vi "Sched and Tubes.vi"(1 "Schedule":T1, 2 "Tube Type":T4, 8 "Error In":errorcluster, 10 "Preselected sched name":string, 11 "Preselected sched":string) -> (0 "Error Out":errorcluster)   [LabVIEW 2023]
uses:
  Schedule.ctl
  Tubes.ctl
  Schedule Name.ctl
  Params.ctl
  QSM - Editor/Controls/State Machine Message.ctl
  QSM - Editor/Controls/Message Queue Element Position.ctl
  QSM - Editor/QSM - Editor.lvlib
panel:
  out "SchedNames":string[](array[string])
  out "SchedNames[]":string[](array[string])
  in  "Tab Control":enum32{"Schedule", "Tubes"}(tab)
  in  "LOAD STEP VAL":bool
  in  "Schedule Name":string
  in  "Sched#":u16(ring) items=["", "Sched1", "Sched2", "Sched3", "Sched4", "Sched5", "Sched6", "Sched7", "Sched8", "Sched9", "Sched10", "Sched11", "Sched12", "Sched13", "Sched14", "Sched15", "Sched16", "Sched17", "Sched18", "Sched19", "Sched20", "Sched21", "Sched22", "Sched23", "Sched24", "Sched25", "Sched26", "Sched27", "Sched28", "Sched29", "Sched30", "Sched31", "Sched32", "Sched33", "Sched34", "Sched35", "Sched36", "Sched37", "Sched38", "Sched39", "Sched40", "Sched41", "Sched42", "Sched43", "Sched44", "Sched45", "Sched46", "Sched47", "Sched48", "Sched49", "Sched50", "Sched51", "Sched52", "Sched53", "Sched54", "Sched55", "Sched56", "Sched57", "Sched58", "Sched59", "Sched60", "Sched61", "Sched62", "Sched63", "Sched64", "Sched65", "Sched66", "Sched67", "Sched68", "Sched69", "Sched70", "Sched71", "Sched72", "Sched73", "Sched74", "Sched75", "Sched76", "Sched77", "Sched78", "Sched79", "Sched80"]
  in  "Load":bool
  out "Schedule Filename":T2
  in  "Save As\nSched":bool
  in  "Zero Sched":bool
  in  "Insert Step":bool
  in  "Delete Step":bool
  in  "Copy Step":bool
  in  "Paste Step":bool
  in  "stop":bool
  in  "stop 2":bool
  in  "Tube Save":bool
  in  "Sched 61-80":T3
  in  "Sched 31-60":T3
  in  "Sched 1-30":T3
  in  "Tube Values":T5
  out "Copied Row":string[](array[string])
  # "--SCHEDULE & TUBE EDITOR--"
  # "** Select tabs at the top to switch between tube & schedule editors"
  # "** If changes are made, please make sure to select the correct schedule and press the 'SAVE AS SCHED' button.\nClosing this screen without saving changes, will result in changes being lost."
  # "** Select tabs at the top to switch between tube & schedule editors"
  # "** To select a tube for editing, double click the desired tube inside the 'Tube Type' Table.\nTo save changed values, the 'SAVE' button must be selected on this screen next to the 'Tube Values' display.\nFailure to save before closing will result in loss of changes."
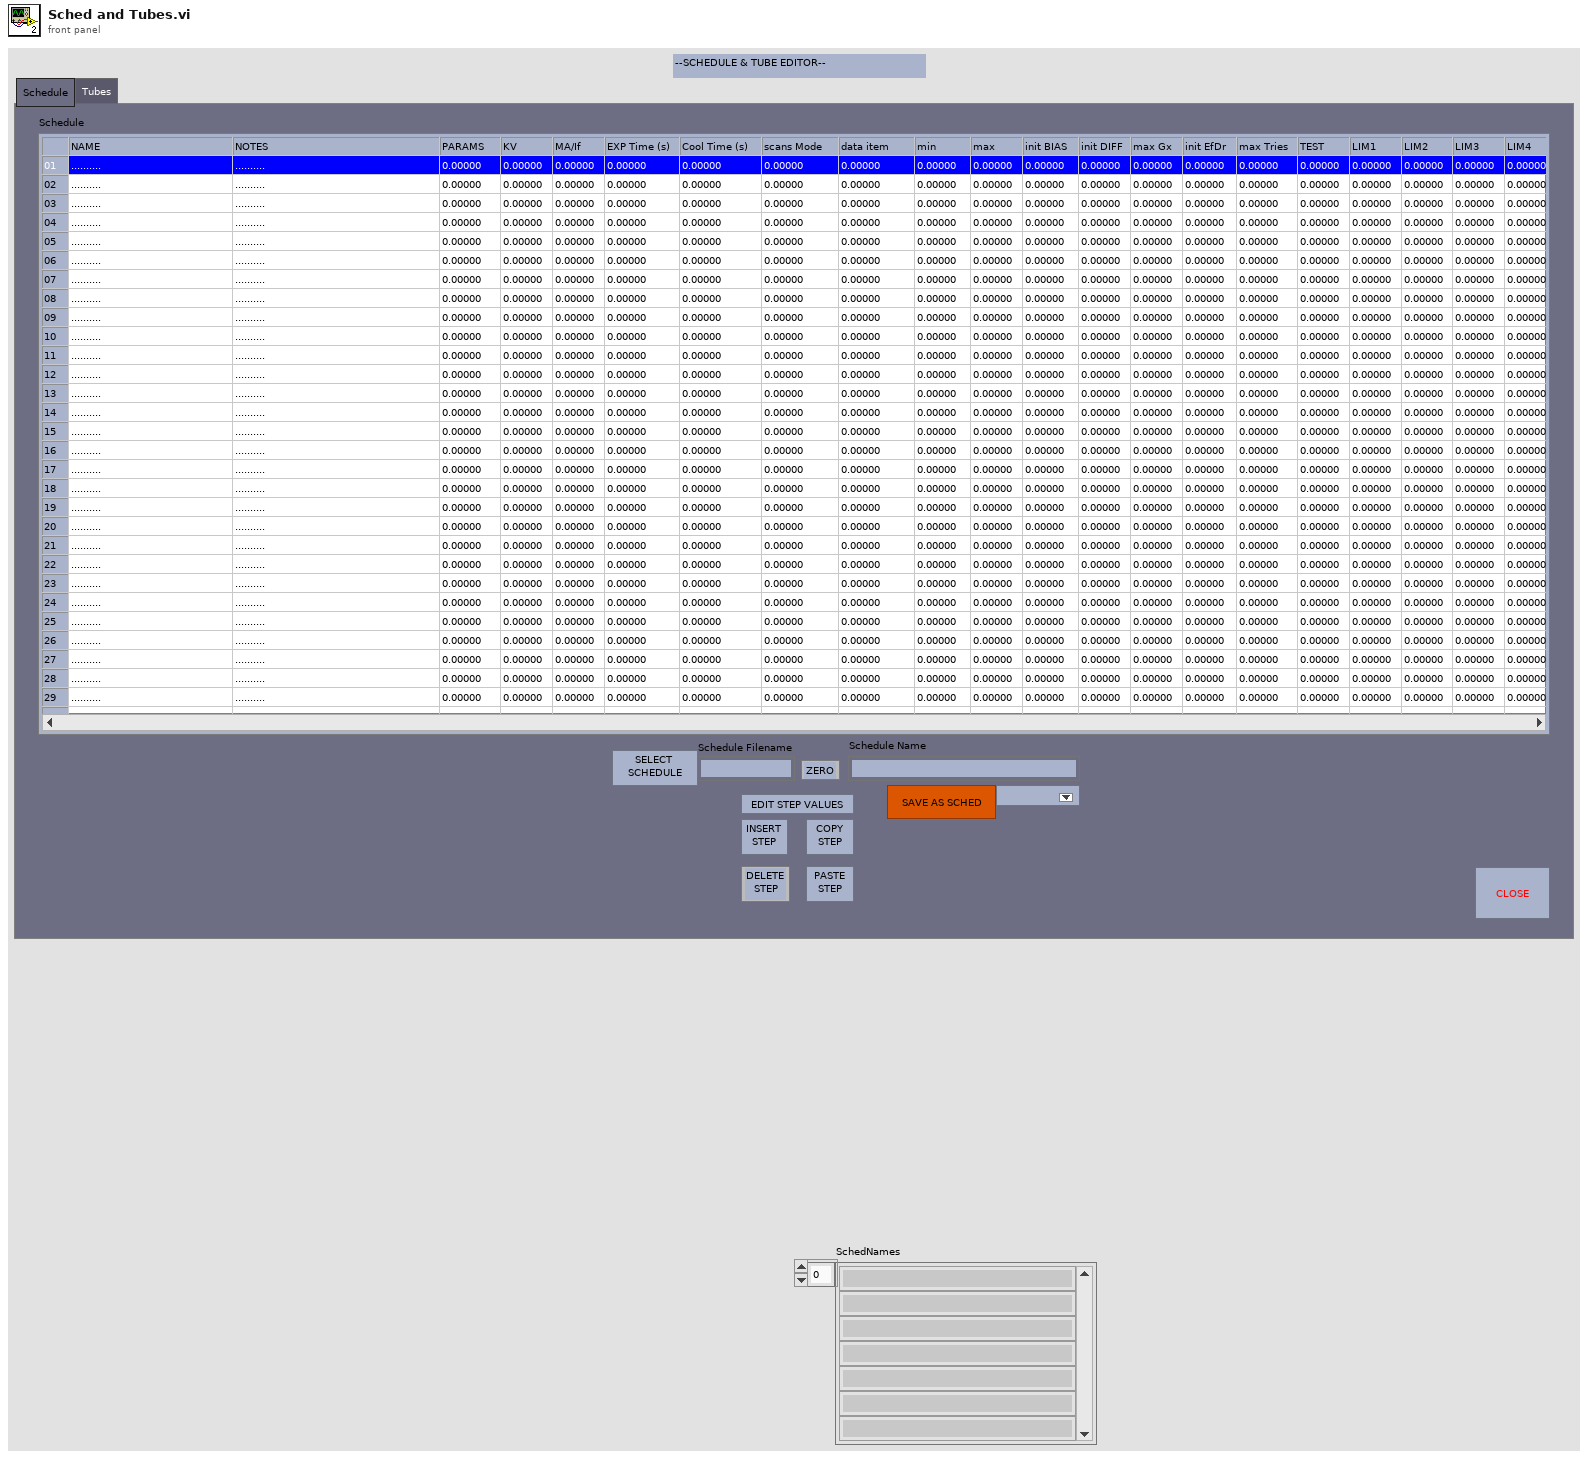
[diagram p1: front panel]
types:
  T1 = typedef "Schedule.ctl" = i32
  T2 = typedef "Schedule Name.ctl" = string
  T3 = typedef "Params.ctl" = cluster{"Boolean":bool, "Boolean 2":bool, "Boolean 3":bool, "Boolean 4":bool, "Boolean 5":bool, "Boolean 6":bool, "Boolean 7":bool, "Boolean 8":bool, "Boolean 9":bool, "Boolean 10":bool, "Boolean 11":bool, "Boolean 12":bool, "Boolean 13":bool, "Boolean 14":bool, "Boolean 15":bool, "Boolean 16":bool, "Boolean 17":bool, "Boolean 18":bool, "Boolean 19":bool, "Boolean 20":bool, "Boolean 21":bool, "Boolean 22":bool, "Boolean 23":bool, "Boolean 24":bool, "Boolean 25":bool, "Boolean 26":bool, "Boolean 27":bool, "Boolean 28":bool, "Boolean 29":bool, "Boolean 30":bool, "Boolean 31":bool, "Boolean 32":bool}
  T4 = typedef "Tubes.ctl" = i32
  T5 = cluster{"Tube Name":string, "T0":dbl, "RTC":dbl, "HS":dbl, "T100":dbl, "AP%":dbl}
  T6 = typedef "QSM - Editor.lvlib/State Machine Message.ctl" = enum16{"Initialize", "Handle Error", "Load", "Zero", "Insert", "Delete", "Copy", "Paste", "Save Sched", "Load Step Vals", "Tubes Tab", "Tube Select", "Tube Save", "Exit"}
  T7 = typedef "QSM - Editor.lvlib/Message Queue Element Position.ctl" = enum16{"Front", "Back"}
  T8 = cluster{"Boolean array[0]":bool, "Boolean array[1]":bool, "Boolean array[2]":bool, "Boolean array[3]":bool, "Boolean array[4]":bool, "Boolean array[5]":bool, "Boolean array[6]":bool, "Boolean array[7]":bool, "Boolean array[8]":bool, "Boolean array[9]":bool, "Boolean array[10]":bool, "Boolean array[11]":bool, "Boolean array[12]":bool, "Boolean array[13]":bool, "Boolean array[14]":bool, "Boolean array[15]":bool, "Boolean array[16]":bool, "Boolean array[17]":bool, "Boolean array[18]":bool, "Boolean array[19]":bool, "Boolean array[20]":bool, "Boolean array[21]":bool, "Boolean array[22]":bool, "Boolean array[23]":bool, "Boolean array[24]":bool, "Boolean array[25]":bool, "Boolean array[26]":bool, "Boolean array[27]":bool, "Boolean array[28]":bool, "Boolean array[29]":bool, "Boolean array[30]":bool, "Boolean array[31]":bool}
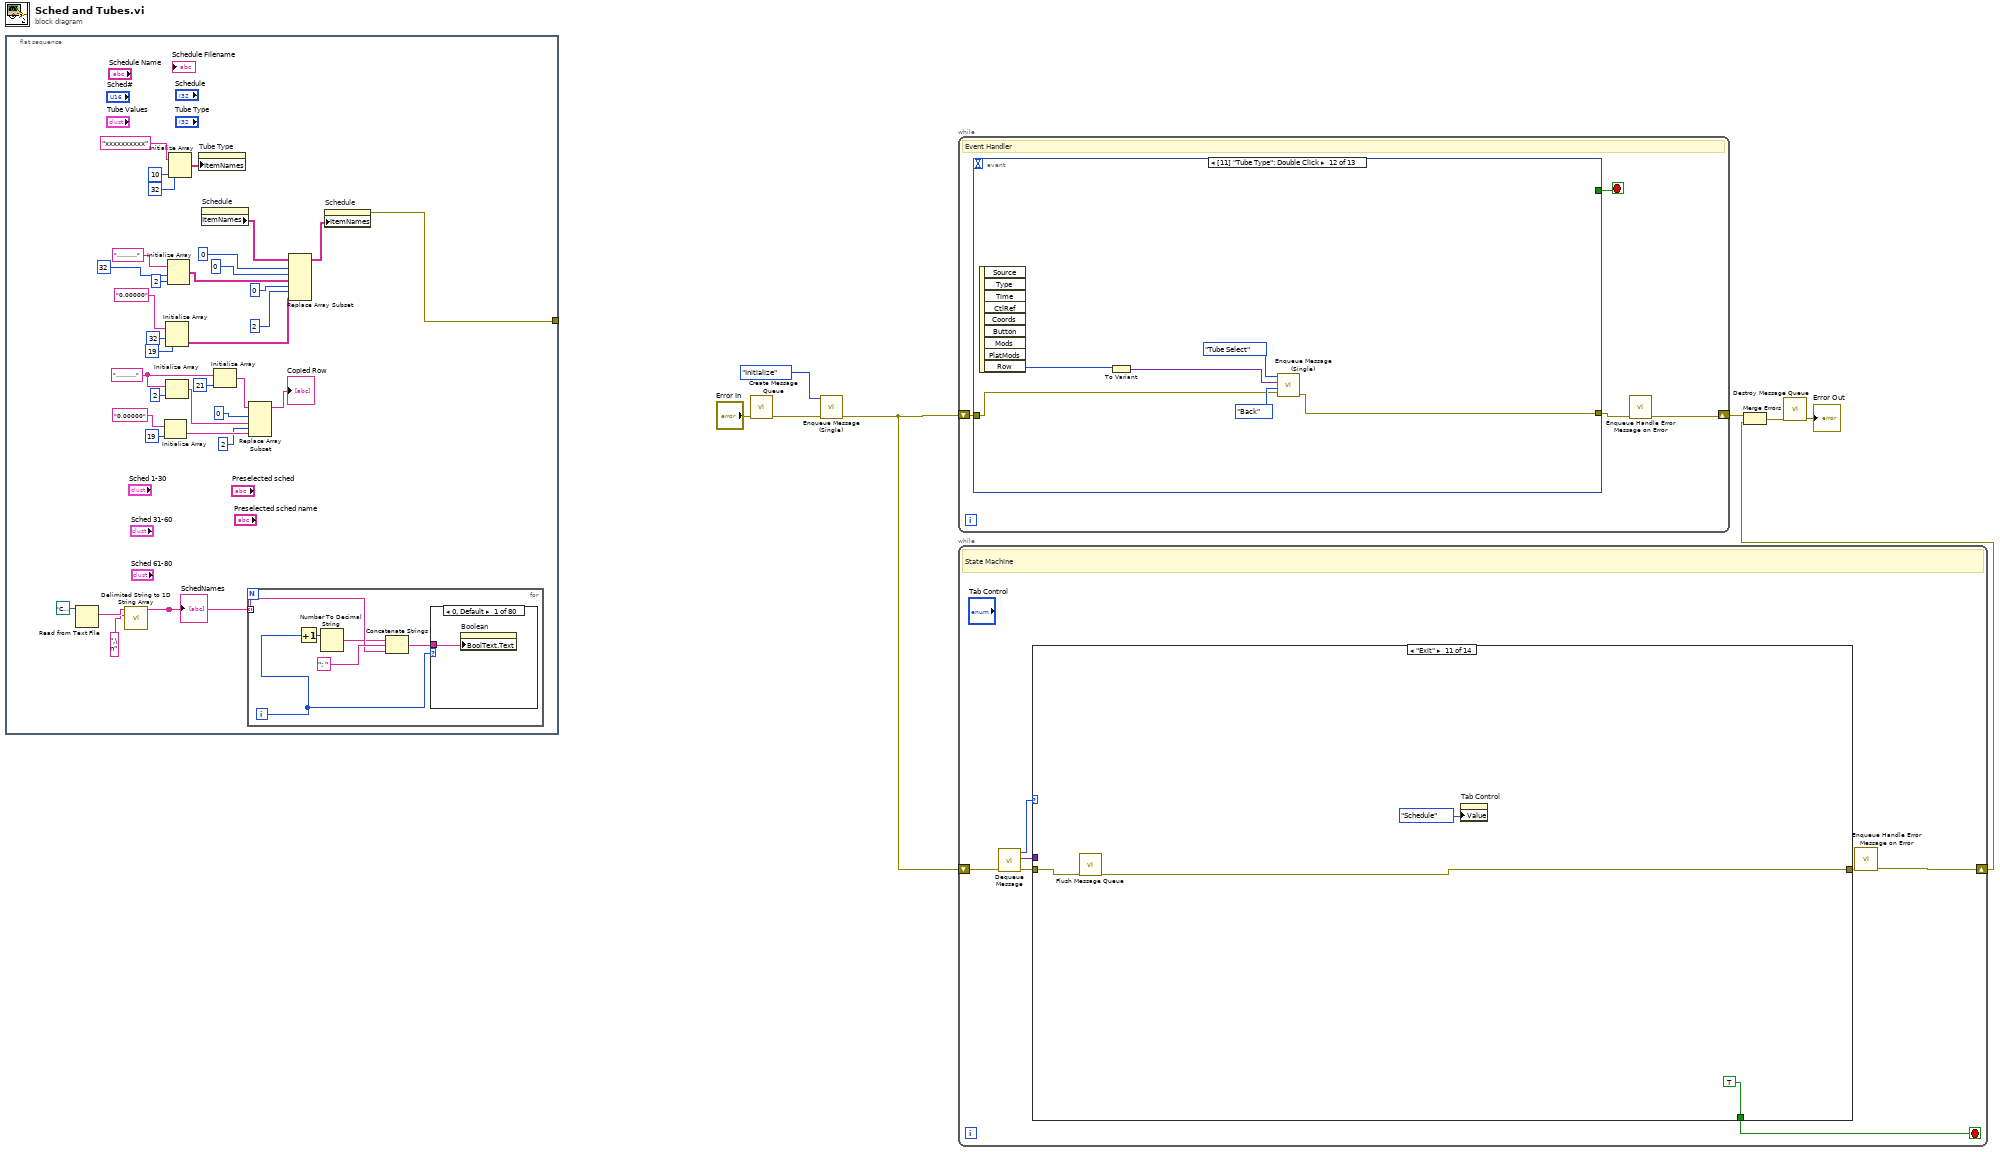
[diagram p0: block diagram]
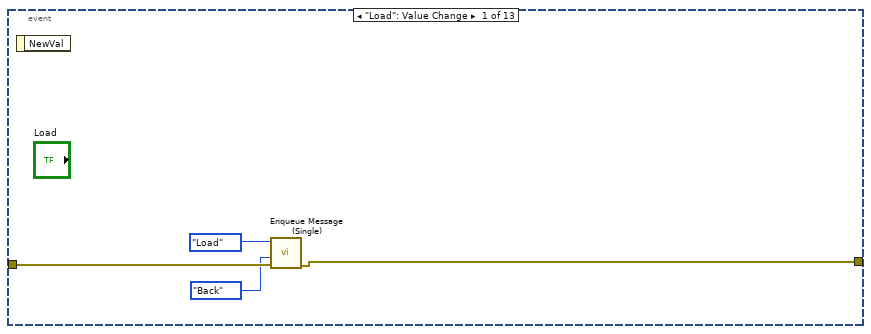
[diagram p2: hidden frame]
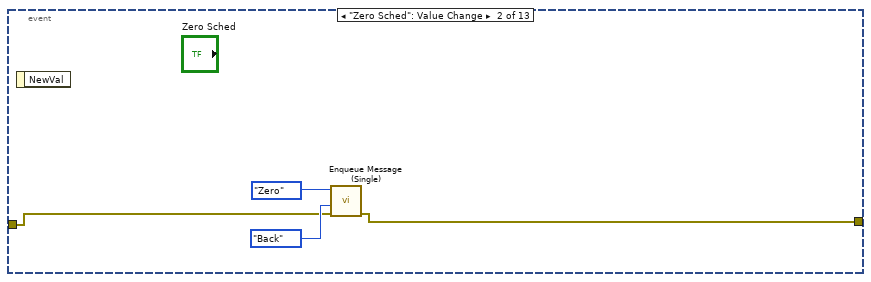
[diagram p3: hidden frame]
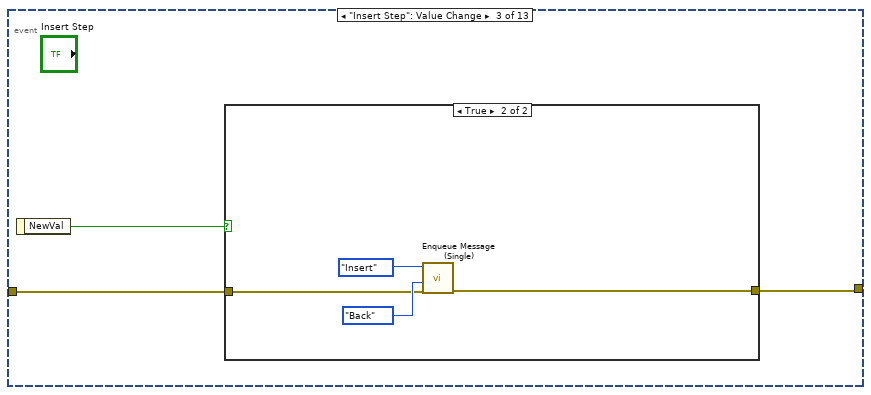
[diagram p4: hidden frame]
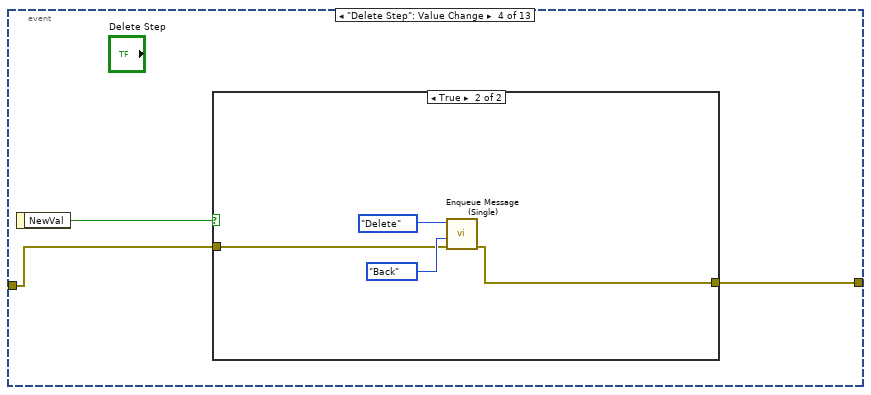
[diagram p6: hidden frame]
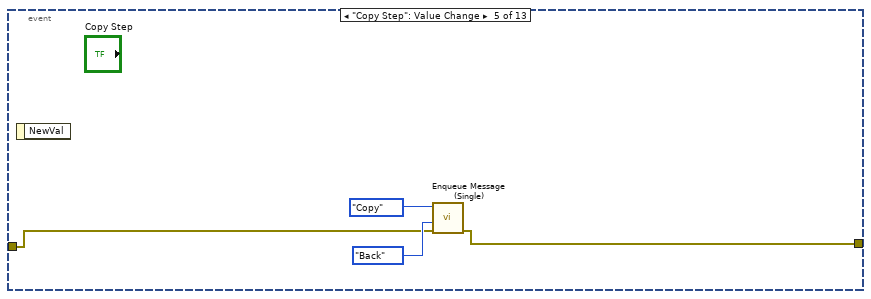
[diagram p8: hidden frame]
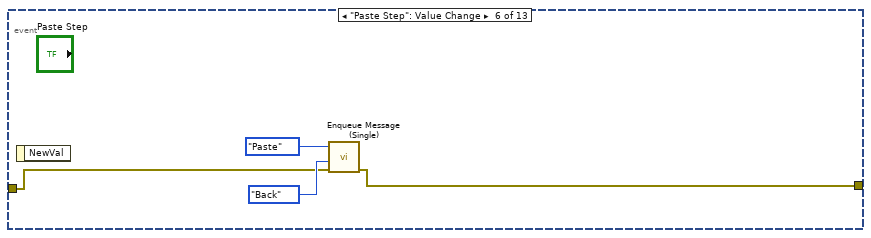
[diagram p9: hidden frame]
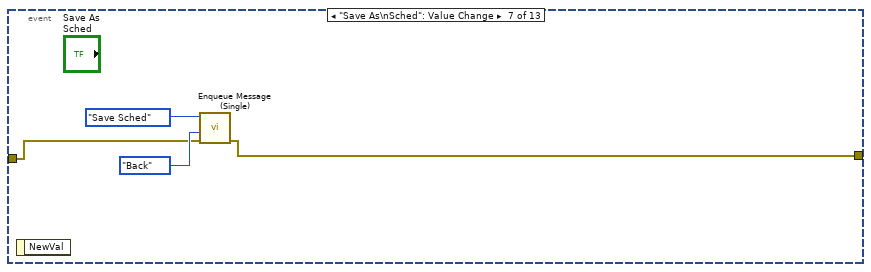
[diagram p10: hidden frame]
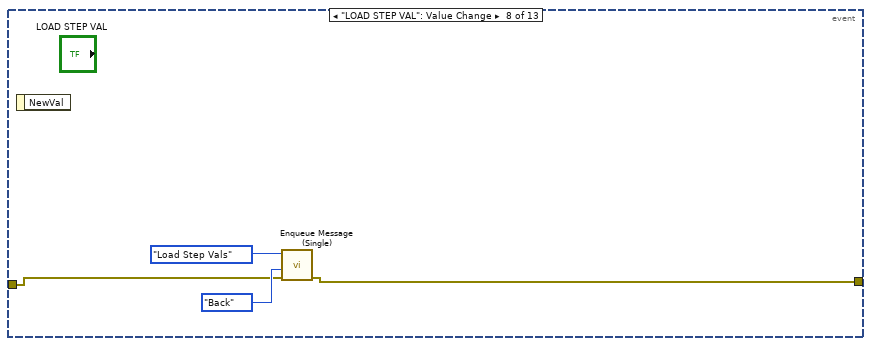
[diagram p11: hidden frame]
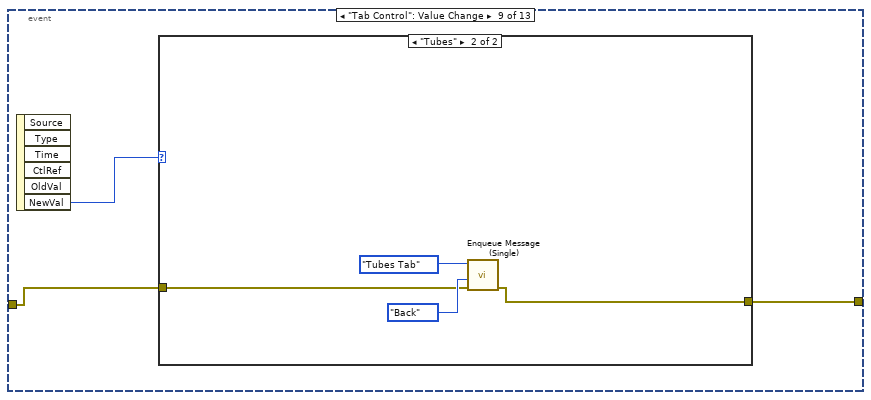
[diagram p12: hidden frame]
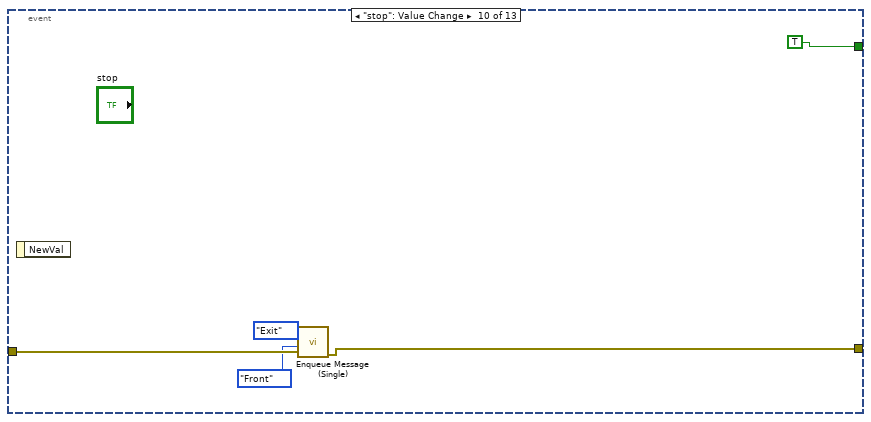
[diagram p14: hidden frame]
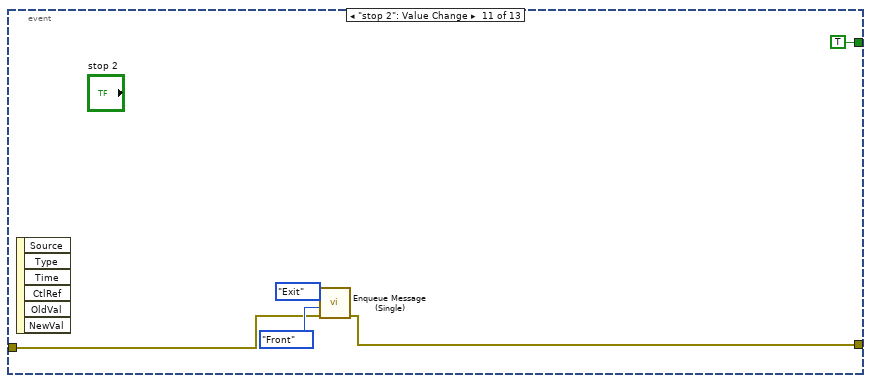
[diagram p15: hidden frame]
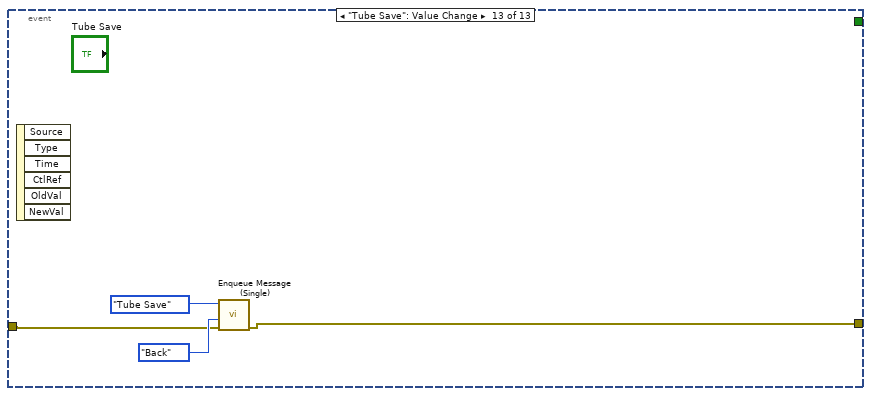
[diagram p16: hidden frame]
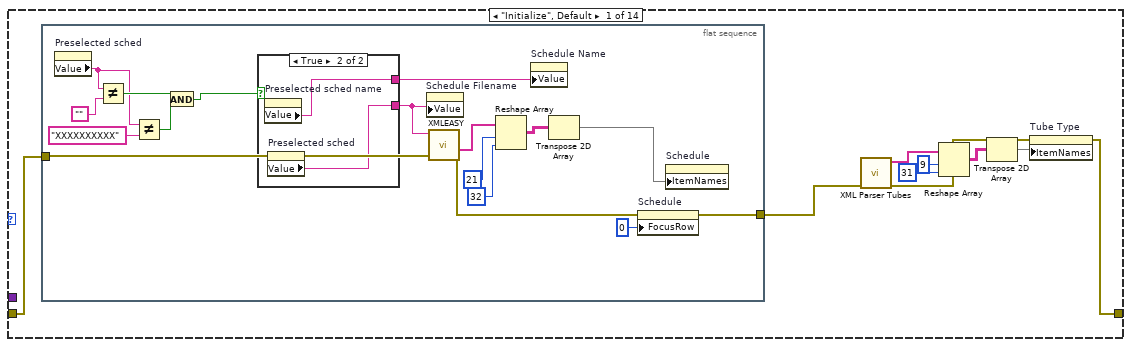
[diagram p17: hidden frame]
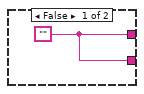
[diagram p18: hidden frame]
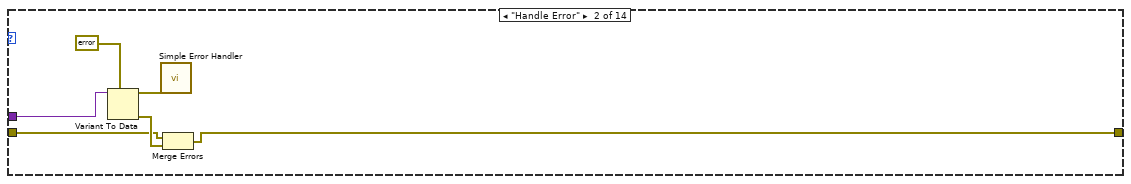
[diagram p19: hidden frame]
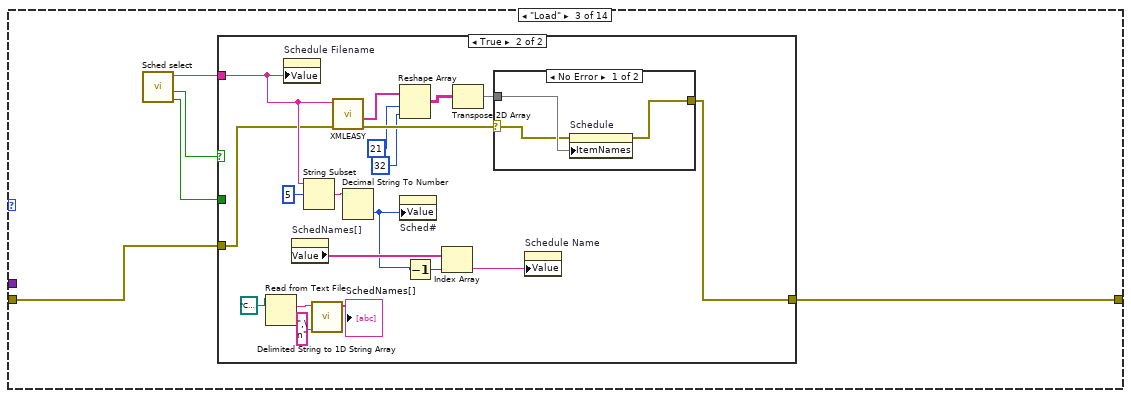
[diagram p20: hidden frame]
diagram:
  n1 = flat-sequence {
    tunnel: [w13] -> _
    frame #0 {
      w19 = ".........."
      n2 = Read from Text File(file (use dialog)=path "C:/Users/Public/Documents/Grid2093/SCHEDS/SchedNames.txt") -> (text=w11:string)  [unwired: 3 in, 3 out]
      n3 = call <vilib>:"Delimited String to 1D String Array.vi"("delimiter"=",\n", "delimited string"=w11) -> ("string array"=w12:string[])  [unwired: 9 in]
      "SchedNames" <- w12
      n4 = Initialize Array("0.00000", 19 ("dimension size")) -> (w23:string[])
      n5 = Initialize Array("0.00000", 32 ("dimension size"), 19 ("dimension size")) -> (w38:string[][])
      n6 = Initialize Array(w19, 2 ("dimension size")) -> (w22:string[])
      n7 = Initialize Array("..........", 32 ("dimension size"), 2 ("dimension size")) -> (w37:string[][])
      n8 = Initialize Array("xxxxxxxxxx", 32 ("dimension size"), 10 ("dimension size")) -> (w39:string[][])
      n9 = property on="Tube Type" class="MCListbox (strict)"("ItemNames"=w39) -> ()  [unwired: 2 in, 2 out]
      n10 = property on="Schedule" class="MCListbox (strict)"() -> ("ItemNames"=w25:string[][])  [unwired: 2 in, 2 out]
      n11 = Initialize Array(w19, 21 ("dimension size")) -> (w24:string[])
      n12 = for {
        tunnel: w12 -> [w47] mode=indexing
        i -> [w44]
        n13 = Increment(x=w44) -> (x+1=w45:i32)
        n14 = Number To Decimal String(number=w45) -> (decimal integer string=w46:string)  [unwired: 1 in]
        n15 = Concatenate Strings(w46, ": " ("string"), w47) -> (w43:string)
        n16 = case shown="0, Default" w44 {
          tunnel: w43 -> [w49 w50 w51 w52 w53 w54 w55 w56 w57 w58 w59 w60 w61 w62 w63 w64 w65 w66 w67 w68 w69 w70 w71 w72 w73 w74 w75 w76 w77 w78 w79 w80 w81 w82 w83 w84 w85 w86 w87 w88 w89 w90 w91 w92 w93 w94 w95 w96 w97 w98 w99 w100 w101 w102 w103 w104 w105 w106 w107 w108 w109 w110 w111 w112 w113 w114 w115 w116 w117 w118 w119 w120 w121 w122 w123 w124 w125 w126 w127 w128]
          frame 0, Default {
            n17 = property on="Boolean" class="Bool (strict)"("BoolText.Text"=w49) -> ()  [unwired: 2 in, 2 out]
          }
          frame 1 {
            n18 = property on="Boolean 2" class="Bool (strict)"("BoolText.Text"=w50) -> ()  [unwired: 2 in, 2 out]
          }
          frame 2 {
            n19 = property on="Boolean 3" class="Bool (strict)"("BoolText.Text"=w51) -> ()  [unwired: 2 in, 2 out]
          }
          frame 3 {
            n20 = property on="Boolean 4" class="Bool (strict)"("BoolText.Text"=w52) -> ()  [unwired: 2 in, 2 out]
          }
          frame 4 {
            n21 = property on="Boolean 5" class="Bool (strict)"("BoolText.Text"=w53) -> ()  [unwired: 2 in, 2 out]
          }
          frame 5 {
            n22 = property on="Boolean 6" class="Bool (strict)"("BoolText.Text"=w54) -> ()  [unwired: 2 in, 2 out]
          }
          frame 6 {
            n23 = property on="Boolean 7" class="Bool (strict)"("BoolText.Text"=w55) -> ()  [unwired: 2 in, 2 out]
          }
          frame 7 {
            n24 = property on="Boolean 8" class="Bool (strict)"("BoolText.Text"=w56) -> ()  [unwired: 2 in, 2 out]
          }
          frame 8 {
            n25 = property on="Boolean 9" class="Bool (strict)"("BoolText.Text"=w57) -> ()  [unwired: 2 in, 2 out]
          }
          frame 9 {
            n26 = property on="Boolean 10" class="Bool (strict)"("BoolText.Text"=w58) -> ()  [unwired: 2 in, 2 out]
          }
          frame 10 {
            n27 = property on="Boolean 11" class="Bool (strict)"("BoolText.Text"=w59) -> ()  [unwired: 2 in, 2 out]
          }
          frame 11 {
            n28 = property on="Boolean 12" class="Bool (strict)"("BoolText.Text"=w60) -> ()  [unwired: 2 in, 2 out]
          }
          frame 12 {
            n29 = property on="Boolean 13" class="Bool (strict)"("BoolText.Text"=w61) -> ()  [unwired: 2 in, 2 out]
          }
          frame 13 {
            n30 = property on="Boolean 14" class="Bool (strict)"("BoolText.Text"=w62) -> ()  [unwired: 2 in, 2 out]
          }
          frame 14 {
            n31 = property on="Boolean 15" class="Bool (strict)"("BoolText.Text"=w63) -> ()  [unwired: 2 in, 2 out]
          }
          frame 15 {
            n32 = property on="Boolean 16" class="Bool (strict)"("BoolText.Text"=w64) -> ()  [unwired: 2 in, 2 out]
          }
          frame 16 {
            n33 = property on="Boolean 17" class="Bool (strict)"("BoolText.Text"=w65) -> ()  [unwired: 2 in, 2 out]
          }
          frame 17 {
            n34 = property on="Boolean 18" class="Bool (strict)"("BoolText.Text"=w66) -> ()  [unwired: 2 in, 2 out]
          }
          frame 18 {
            n35 = property on="Boolean 19" class="Bool (strict)"("BoolText.Text"=w67) -> ()  [unwired: 2 in, 2 out]
          }
          frame 19 {
            n36 = property on="Boolean 20" class="Bool (strict)"("BoolText.Text"=w68) -> ()  [unwired: 2 in, 2 out]
          }
          frame 20 {
            n37 = property on="Boolean 21" class="Bool (strict)"("BoolText.Text"=w69) -> ()  [unwired: 2 in, 2 out]
          }
          frame 21 {
            n38 = property on="Boolean 22" class="Bool (strict)"("BoolText.Text"=w70) -> ()  [unwired: 2 in, 2 out]
          }
          frame 22 {
            n39 = property on="Boolean 23" class="Bool (strict)"("BoolText.Text"=w71) -> ()  [unwired: 2 in, 2 out]
          }
          frame 23 {
            n40 = property on="Boolean 24" class="Bool (strict)"("BoolText.Text"=w72) -> ()  [unwired: 2 in, 2 out]
          }
          frame 24 {
            n41 = property on="Boolean 25" class="Bool (strict)"("BoolText.Text"=w73) -> ()  [unwired: 2 in, 2 out]
          }
          frame 25 {
            n42 = property on="Boolean 26" class="Bool (strict)"("BoolText.Text"=w74) -> ()  [unwired: 2 in, 2 out]
          }
          frame 26 {
            n43 = property on="Boolean 27" class="Bool (strict)"("BoolText.Text"=w75) -> ()  [unwired: 2 in, 2 out]
          }
          frame 27 {
            n44 = property on="Boolean 28" class="Bool (strict)"("BoolText.Text"=w76) -> ()  [unwired: 2 in, 2 out]
          }
          frame 28 {
            n45 = property on="Boolean 29" class="Bool (strict)"("BoolText.Text"=w77) -> ()  [unwired: 2 in, 2 out]
          }
          frame 29 {
            n46 = property on="Boolean 30" class="Bool (strict)"("BoolText.Text"=w78) -> ()  [unwired: 2 in, 2 out]
          }
          frame 30 {
            n47 = property on="Boolean" class="Bool (strict)"("BoolText.Text"=w79) -> ()  [unwired: 2 in, 2 out]
          }
          frame 31 {
            n48 = property on="Boolean 2" class="Bool (strict)"("BoolText.Text"=w80) -> ()  [unwired: 2 in, 2 out]
          }
          frame 32 {
            n49 = property on="Boolean 3" class="Bool (strict)"("BoolText.Text"=w81) -> ()  [unwired: 2 in, 2 out]
          }
          frame 33 {
            n50 = property on="Boolean 4" class="Bool (strict)"("BoolText.Text"=w82) -> ()  [unwired: 2 in, 2 out]
          }
          frame 34 {
            n51 = property on="Boolean 5" class="Bool (strict)"("BoolText.Text"=w83) -> ()  [unwired: 2 in, 2 out]
          }
          frame 35 {
            n52 = property on="Boolean 6" class="Bool (strict)"("BoolText.Text"=w84) -> ()  [unwired: 2 in, 2 out]
          }
          frame 36 {
            n53 = property on="Boolean 7" class="Bool (strict)"("BoolText.Text"=w85) -> ()  [unwired: 2 in, 2 out]
          }
          frame 37 {
            n54 = property on="Boolean 8" class="Bool (strict)"("BoolText.Text"=w86) -> ()  [unwired: 2 in, 2 out]
          }
          frame 38 {
            n55 = property on="Boolean 9" class="Bool (strict)"("BoolText.Text"=w87) -> ()  [unwired: 2 in, 2 out]
          }
          frame 39 {
            n56 = property on="Boolean 10" class="Bool (strict)"("BoolText.Text"=w88) -> ()  [unwired: 2 in, 2 out]
          }
          frame 40 {
            n57 = property on="Boolean 11" class="Bool (strict)"("BoolText.Text"=w89) -> ()  [unwired: 2 in, 2 out]
          }
          frame 41 {
            n58 = property on="Boolean 12" class="Bool (strict)"("BoolText.Text"=w90) -> ()  [unwired: 2 in, 2 out]
          }
          frame 42 {
            n59 = property on="Boolean 13" class="Bool (strict)"("BoolText.Text"=w91) -> ()  [unwired: 2 in, 2 out]
          }
          frame 43 {
            n60 = property on="Boolean 14" class="Bool (strict)"("BoolText.Text"=w92) -> ()  [unwired: 2 in, 2 out]
          }
          frame 44 {
            n61 = property on="Boolean 15" class="Bool (strict)"("BoolText.Text"=w93) -> ()  [unwired: 2 in, 2 out]
          }
          frame 45 {
            n62 = property on="Boolean 16" class="Bool (strict)"("BoolText.Text"=w94) -> ()  [unwired: 2 in, 2 out]
          }
          frame 46 {
            n63 = property on="Boolean 17" class="Bool (strict)"("BoolText.Text"=w95) -> ()  [unwired: 2 in, 2 out]
          }
          frame 47 {
            n64 = property on="Boolean 18" class="Bool (strict)"("BoolText.Text"=w96) -> ()  [unwired: 2 in, 2 out]
          }
          frame 48 {
            n65 = property on="Boolean 19" class="Bool (strict)"("BoolText.Text"=w97) -> ()  [unwired: 2 in, 2 out]
          }
          frame 49 {
            n66 = property on="Boolean 20" class="Bool (strict)"("BoolText.Text"=w98) -> ()  [unwired: 2 in, 2 out]
          }
          frame 50 {
            n67 = property on="Boolean 21" class="Bool (strict)"("BoolText.Text"=w99) -> ()  [unwired: 2 in, 2 out]
          }
          frame 51 {
            n68 = property on="Boolean 22" class="Bool (strict)"("BoolText.Text"=w100) -> ()  [unwired: 2 in, 2 out]
          }
          frame 52 {
            n69 = property on="Boolean 23" class="Bool (strict)"("BoolText.Text"=w101) -> ()  [unwired: 2 in, 2 out]
          }
          frame 53 {
            n70 = property on="Boolean 24" class="Bool (strict)"("BoolText.Text"=w102) -> ()  [unwired: 2 in, 2 out]
          }
          frame 54 {
            n71 = property on="Boolean 25" class="Bool (strict)"("BoolText.Text"=w103) -> ()  [unwired: 2 in, 2 out]
          }
          frame 55 {
            n72 = property on="Boolean 26" class="Bool (strict)"("BoolText.Text"=w104) -> ()  [unwired: 2 in, 2 out]
          }
          frame 56 {
            n73 = property on="Boolean 27" class="Bool (strict)"("BoolText.Text"=w105) -> ()  [unwired: 2 in, 2 out]
          }
          frame 57 {
            n74 = property on="Boolean 28" class="Bool (strict)"("BoolText.Text"=w106) -> ()  [unwired: 2 in, 2 out]
          }
          frame 58 {
            n75 = property on="Boolean 29" class="Bool (strict)"("BoolText.Text"=w107) -> ()  [unwired: 2 in, 2 out]
          }
          frame 59 {
            n76 = property on="Boolean 30" class="Bool (strict)"("BoolText.Text"=w108) -> ()  [unwired: 2 in, 2 out]
          }
          frame 60 {
            n77 = property on="Boolean" class="Bool (strict)"("BoolText.Text"=w109) -> ()  [unwired: 2 in, 2 out]
          }
          frame 61 {
            n78 = property on="Boolean 2" class="Bool (strict)"("BoolText.Text"=w110) -> ()  [unwired: 2 in, 2 out]
          }
          frame 62 {
            n79 = property on="Boolean 3" class="Bool (strict)"("BoolText.Text"=w111) -> ()  [unwired: 2 in, 2 out]
          }
          frame 63 {
            n80 = property on="Boolean 4" class="Bool (strict)"("BoolText.Text"=w112) -> ()  [unwired: 2 in, 2 out]
          }
          frame 64 {
            n81 = property on="Boolean 5" class="Bool (strict)"("BoolText.Text"=w113) -> ()  [unwired: 2 in, 2 out]
          }
          frame 65 {
            n82 = property on="Boolean 6" class="Bool (strict)"("BoolText.Text"=w114) -> ()  [unwired: 2 in, 2 out]
          }
          frame 66 {
            n83 = property on="Boolean 7" class="Bool (strict)"("BoolText.Text"=w115) -> ()  [unwired: 2 in, 2 out]
          }
          frame 67 {
            n84 = property on="Boolean 8" class="Bool (strict)"("BoolText.Text"=w116) -> ()  [unwired: 2 in, 2 out]
          }
          frame 68 {
            n85 = property on="Boolean 9" class="Bool (strict)"("BoolText.Text"=w117) -> ()  [unwired: 2 in, 2 out]
          }
          frame 69 {
            n86 = property on="Boolean 10" class="Bool (strict)"("BoolText.Text"=w118) -> ()  [unwired: 2 in, 2 out]
          }
          frame 70 {
            n87 = property on="Boolean 11" class="Bool (strict)"("BoolText.Text"=w119) -> ()  [unwired: 2 in, 2 out]
          }
          frame 71 {
            n88 = property on="Boolean 12" class="Bool (strict)"("BoolText.Text"=w120) -> ()  [unwired: 2 in, 2 out]
          }
          frame 72 {
            n89 = property on="Boolean 13" class="Bool (strict)"("BoolText.Text"=w121) -> ()  [unwired: 2 in, 2 out]
          }
          frame 73 {
            n90 = property on="Boolean 14" class="Bool (strict)"("BoolText.Text"=w122) -> ()  [unwired: 2 in, 2 out]
          }
          frame 74 {
            n91 = property on="Boolean 15" class="Bool (strict)"("BoolText.Text"=w123) -> ()  [unwired: 2 in, 2 out]
          }
          frame 75 {
            n92 = property on="Boolean 16" class="Bool (strict)"("BoolText.Text"=w124) -> ()  [unwired: 2 in, 2 out]
          }
          frame 76 {
            n93 = property on="Boolean 17" class="Bool (strict)"("BoolText.Text"=w125) -> ()  [unwired: 2 in, 2 out]
          }
          frame 77 {
            n94 = property on="Boolean 18" class="Bool (strict)"("BoolText.Text"=w126) -> ()  [unwired: 2 in, 2 out]
          }
          frame 78 {
            n95 = property on="Boolean 19" class="Bool (strict)"("BoolText.Text"=w127) -> ()  [unwired: 2 in, 2 out]
          }
          frame 79 {
            n96 = property on="Boolean 20" class="Bool (strict)"("BoolText.Text"=w128) -> ()  [unwired: 2 in, 2 out]
          }
        }
      }
      n97 = Replace Array Subset(array=w24, new element #1=w22, index #1=0 ("index"), new element #2=w23, index #2=2 ("index")) -> (→"Copied Row":string[])
      n98 = Replace Array Subset(array=w25, new element #1=w37, index (row) #1=0 ("index"), index (col) #1=0 ("disabled index (col)"), new element #2=w38, index (row) #2=0 ("index"), index (col) #2=2 ("disabled index (col)")) -> (w27:string[][])
      n99 = property on="Schedule" class="MCListbox (strict)"("ItemNames"=w27) -> (error out=w13:errorcluster)  [unwired: 2 in, 1 out]
    }
  }
  n100 = call "Create Message Queue.vi"("Error In"="Error In") -> ("Error Out"=w8:errorcluster)  [unwired: 10 in]
  n101 = call "Enqueue Message (Single).vi"("Error In"=w8, "State Machine Message"=State_Machine_Message."Initialize") -> ("Error Out"=w4:errorcluster)  [unwired: 9 in]
  n102 = while {
    shift-right: [w129] -> w6
    shift-left: w4 -> [w131]
    stop <- w132 stop-if-true
    # "Event Handler"
    n103 = event shown="[11] \"Tube Type\": Double Click" {
      selector: _ -> [_ _ _ _ _ _ _ _ _ _ _ _ _]
      dyn-events: _ -> [_ _ _ _ _ _ _ _ _ _ _ _ _]
      timeout: _ -> [_ _ _ _ _ _ _ _ _ _ _ _ _]
      tunnel: [_ _ _ _ _ _ _ _ _ TRUE TRUE _ _] -> w132
      tunnel: w131 -> [w136 w138 w142 w150 w158 w162 w166 w170 w174 w184 w187 w194 w198]
      tunnel: [w133 w137 w141 w149 w157 w161 w165 w169 w173 w181 w186 w191 w197] -> w130
      event "Load": Value Change {
        n104 = event-data() -> ()  [unwired: 1 in, 1 out]
        n105 = call "Enqueue Message (Single).vi"("Error In"=w136, "Message Position"=Message_Queue_Element_Position."Back", "State Machine Message"=State_Machine_Message."Load") -> ("Error Out"=w133:errorcluster)  [unwired: 8 in]
      }
      event "Zero Sched": Value Change {
        n106 = event-data() -> ()  [unwired: 1 in, 1 out]
        n107 = call "Enqueue Message (Single).vi"("Error In"=w138, "Message Position"=Message_Queue_Element_Position."Back", "State Machine Message"=State_Machine_Message."Zero") -> ("Error Out"=w137:errorcluster)  [unwired: 8 in]
      }
      event "Insert Step": Value Change {
        n108 = event-data() -> ("NewVal"=w143:bool)  [unwired: 1 in]
        n109 = case shown="True" w143 {
          tunnel: w142 -> [w144 w146]
          tunnel: [w144 w145] -> w141
          frame False {
          }
          frame True {
            n110 = call "Enqueue Message (Single).vi"("Error In"=w146, "Message Position"=Message_Queue_Element_Position."Back", "State Machine Message"=State_Machine_Message."Insert") -> ("Error Out"=w145:errorcluster)  [unwired: 8 in]
          }
        }
      }
      event "Delete Step": Value Change {
        n111 = event-data() -> ("NewVal"=w151:bool)  [unwired: 1 in]
        n112 = case shown="True" w151 {
          tunnel: w150 -> [w152 w154]
          tunnel: [w152 w153] -> w149
          frame False {
          }
          frame True {
            n113 = call "Enqueue Message (Single).vi"("Error In"=w154, "Message Position"=Message_Queue_Element_Position."Back", "State Machine Message"=State_Machine_Message."Delete") -> ("Error Out"=w153:errorcluster)  [unwired: 8 in]
          }
        }
      }
      event "Copy Step": Value Change {
        n114 = event-data() -> ()  [unwired: 1 in, 1 out]
        n115 = call "Enqueue Message (Single).vi"("Error In"=w158, "Message Position"=Message_Queue_Element_Position."Back", "State Machine Message"=State_Machine_Message."Copy") -> ("Error Out"=w157:errorcluster)  [unwired: 8 in]
      }
      event "Paste Step": Value Change {
        n116 = event-data() -> ()  [unwired: 1 in, 1 out]
        n117 = call "Enqueue Message (Single).vi"("Error In"=w162, "Message Position"=Message_Queue_Element_Position."Back", "State Machine Message"=State_Machine_Message."Paste") -> ("Error Out"=w161:errorcluster)  [unwired: 8 in]
      }
      event "Save As\nSched": Value Change {
        n118 = event-data() -> ()  [unwired: 1 in, 1 out]
        n119 = call "Enqueue Message (Single).vi"("Error In"=w166, "Message Position"=Message_Queue_Element_Position."Back", "State Machine Message"=State_Machine_Message."Save Sched") -> ("Error Out"=w165:errorcluster)  [unwired: 8 in]
      }
      event "LOAD STEP VAL": Value Change {
        n120 = event-data() -> ()  [unwired: 1 in, 1 out]
        n121 = call "Enqueue Message (Single).vi"("Error In"=w170, "Message Position"=Message_Queue_Element_Position."Back", "State Machine Message"=State_Machine_Message."Load Step Vals") -> ("Error Out"=w169:errorcluster)  [unwired: 8 in]
      }
      event "Tab Control": Value Change {
        n122 = event-data() -> ("NewVal"=w175:enum32{"Schedule", "Tubes"})  [unwired: 1 in, 5 out]
        n123 = case shown="\"Tubes\"" w175 {
          tunnel: w174 -> [w176 w178]
          tunnel: [w176 w177] -> w173
          frame "Schedule", Default {
          }
          frame "Tubes" {
            n124 = call "Enqueue Message (Single).vi"("Error In"=w178, "Message Position"=Message_Queue_Element_Position."Back", "State Machine Message"=State_Machine_Message."Tubes Tab") -> ("Error Out"=w177:errorcluster)  [unwired: 8 in]
          }
        }
      }
      event "stop": Value Change {
        n125 = event-data() -> ()  [unwired: 1 in, 1 out]
        n126 = call "Enqueue Message (Single).vi"("Error In"=w184, "Message Position"=Message_Queue_Element_Position."Front", "State Machine Message"=State_Machine_Message."Exit") -> ("Error Out"=w181:errorcluster)  [unwired: 8 in]
      }
      event "stop 2": Value Change {
        n127 = event-data() -> ()  [unwired: 1 in, 6 out]
        n128 = call "Enqueue Message (Single).vi"("Error In"=w187, "Message Position"=Message_Queue_Element_Position."Front", "State Machine Message"=State_Machine_Message."Exit") -> ("Error Out"=w186:errorcluster)  [unwired: 8 in]
      }
      event Double Click {
        n129 = event-data() -> ("Row"=w193:i32)  [unwired: 1 in, 8 out]
        n130 = To Variant(anything=w193) -> (Variant=w192:variant)
        n131 = call "Enqueue Message (Single).vi"("Error In"=w194, "Message Position"=Message_Queue_Element_Position."Back", "Data"=w192, "State Machine Message"=State_Machine_Message."Tube Select") -> ("Error Out"=w191:errorcluster)  [unwired: 7 in]
      }
      event "Tube Save": Value Change {
        n132 = event-data() -> ()  [unwired: 1 in, 6 out]
        n133 = call "Enqueue Message (Single).vi"("Error In"=w198, "Message Position"=Message_Queue_Element_Position."Back", "State Machine Message"=State_Machine_Message."Tube Save") -> ("Error Out"=w197:errorcluster)  [unwired: 8 in]
      }
    }
    n134 = call "Enqueue Handle Error Message on Error.vi"("Error In"=w130) -> ("Error Out"=w129:errorcluster)  [unwired: 10 in]
  }
  n135 = while {
    shift-right: [w202] -> w3
    shift-left: w4 -> [w207]
    stop <- w201 stop-if-true
    # "State Machine"
    n136 = call "Dequeue Message.vi"("Error In"=w207) -> ("Error Out"=w205:errorcluster, "Data"=w204:variant, "State Machine Message"=w206:T6)  [unwired: 8 in]
    n137 = case shown="\"Exit\"" w206 {
      tunnel: w205 -> [w210 w240 w243 w272 w287 w302 w321 w325 w336 w357 w375 w383 w395 w461]
      tunnel: w204 -> [_ w242 _ _ _ _ _ _ _ _ _ _ w394 _]
      tunnel: [w209 w237 w244 w272 w287 w302 w321 w325 w335 w357 w374 w377 w391 w460] -> w203
      tunnel: [_ _ _ _ _ _ _ _ _ _ TRUE _ _ _] -> w201
      frame "Initialize", Default {
        n138 = flat-sequence {
          tunnel: w210 -> [w228]
          tunnel: [w217] -> w208
          frame #0 {
            n139 = property on="Preselected sched" class="Str"() -> ("Value"=w222:string)  [unwired: 2 in, 2 out]
            n140 = Not Equal?(x=w222, y="") -> (x != y?=w224:bool)
            n141 = Not Equal?(x=w222, y="XXXXXXXXXX") -> (x != y?=w223:bool)
            n142 = And(x=w224, y=w223) -> (x .and. y?=w220:bool)
            n143 = case shown="True" w220 {
              tunnel: [w234 w236] -> w226
              tunnel: [w234 w235] -> w225
              frame False {
                w234 = "" ("Schedule Filename")
              }
              frame True {
                n144 = property on="Preselected sched name" class="Str"() -> ("Value"=w236:string)  [unwired: 2 in, 2 out]
                n145 = property on="Preselected sched" class="Str"() -> ("Value"=w235:string)  [unwired: 2 in, 2 out]
              }
            }
            n146 = property on="Schedule Filename" class="Str (strict)"("Value"=w225) -> ()  [unwired: 2 in, 2 out]
            n147 = call "XMLEASY.vi"("error in (no error)"=w228, "Schedule Filename"=w225) -> ("error out"=w219:errorcluster, "Sched Tag Vals (1D)"=w232:string[])  [unwired: 6 in, 2 out]
            n148 = Reshape Array(w232, 21 ("dimension size"), 32 ("dimension size")) -> (w231:string[][])
            n149 = property on="Schedule Name" class="Str"("Value"=w226) -> ()  [unwired: 2 in, 2 out]
            n150 = Transpose 2D Array(2D array=w231) -> (transposed array=w230:string[][])
            n151 = property on="Schedule" class="MCListbox (strict)"(error in=w219, "FocusRow"=0 ("Focus Row")) -> (error out=w217:errorcluster)  [unwired: 1 in, 1 out]
            n152 = property on="Schedule" class="MCListbox (strict)"("ItemNames"=w230) -> ()  [unwired: 2 in, 2 out]
          }
        }
        n153 = call "XML Parser Tubes.vi"("error in (no error)"=w208) -> ("error out"=w216:errorcluster, "output array"=w215:string[])  [unwired: 9 in]
        n154 = Reshape Array(w215, 9 ("dimension size"), 31 ("dimension size")) -> (w214:string[][])
        n155 = Transpose 2D Array(2D array=w214) -> (transposed array=w213:string[][])
        n156 = property on="Tube Type" class="MCListbox (strict)"(error in=w216, "ItemNames"=w213) -> (error out=w209:errorcluster)  [unwired: 1 in, 1 out]
      }
      frame "Handle Error" {
        n157 = Variant To Data(type=errorcluster {"status"=FALSE, "code"=0, "source"=""}, Variant=w242) -> (data=w239:errorcluster, error out=w241:errorcluster)  [unwired: 1 in]
        n158 = call <vilib>:"Simple Error Handler.vi"("error in (no error)"=w239) -> ()  [unwired: 4 in, 5 out]
        n159 = Merge Errors(w240, w241) -> (w237:errorcluster)
      }
      frame "Load" {
        n160 = call "Sched select.vi"() -> ("Close"=w247:bool, "Load"=w246:bool, "selected sched"=w245:string)  [unwired: 9 in]
        n161 = case shown="True" w246 {
          tunnel: w245 -> [_ w267]
          tunnel: w247 -> [_ _]
          tunnel: [w248 w250] -> w244
          tunnel: w243 -> [w248 w249]
          frame False {
          }
          frame True {
            n162 = Read from Text File(file (use dialog)=path "C:/Users/Public/Documents/Grid2093/SCHEDS/SchedNames.txt" ("path")) -> (text=w253:string)  [unwired: 3 in, 3 out]
            n163 = property on="Schedule Filename" class="Str (strict)"("Value"=w267) -> ()  [unwired: 2 in, 2 out]
            n164 = property on="SchedNames[]" class="Arr (strict)"() -> ("Value"=w258:string[])  [unwired: 2 in, 2 out]
            n165 = String Subset(string=w267, offset (0)=5) -> (substring=w260:string)  [unwired: 1 in]
            n166 = call <vilib>:"Delimited String to 1D String Array.vi"("delimiter"=",\n", "delimited string"=w253) -> ("string array"=→"SchedNames[]":string[])  [unwired: 9 in]
            n167 = call "XMLEASY.vi"("error in (no error)"=w249, "Schedule Filename"=w267) -> ("error out"=w266:errorcluster, "Sched Tag Vals (1D)"=w263:string[])  [unwired: 6 in, 2 out]
            n168 = Decimal String To Number(string=w260) -> (number=w255:i32)  [unwired: 2 in, 1 out]
            n169 = Reshape Array(w263, 21 ("dimension size"), 32 ("dimension size")) -> (w262:string[][])
            n170 = property on="Sched#" class="Ring (strict)"("Value"=w255) -> ()  [unwired: 2 in, 2 out]
            n171 = Decrement(x=w255) -> (x-1=w256:i32)
            n172 = Index Array(array=w258, index=w256) -> (element=w257:string)
            n173 = Transpose 2D Array(2D array=w262) -> (transposed array=w261:string[][])
            n174 = case shown="No Error" w266 {
              selector: w266 -> [w269 w271]
              tunnel: [w268 w271] -> w250
              tunnel: w261 -> [w270 _]
              frame No Error {
                n175 = property on="Schedule" class="MCListbox (strict)"(error in=w269, "ItemNames"=w270) -> (error out=w268:errorcluster)  [unwired: 1 in, 1 out]
              }
              frame Error {
              }
            }
            n176 = property on="Schedule Name" class="Str"("Value"=w257) -> ()  [unwired: 2 in, 2 out]
          }
        }
      }
      frame "Zero" {
        n177 = Initialize Array("..........", 32 ("dimension size"), 2 ("dimension size")) -> (w284:string[][])
        n178 = Initialize Array("0.00000", 32 ("dimension size"), 19 ("dimension size")) -> (w285:string[][])
        n179 = property on="Schedule" class="MCListbox (strict)"() -> ("ItemNames"=w283:string[][])  [unwired: 2 in, 2 out]
        n180 = Replace Array Subset(array=w283, new element #1=w284, index (row) #1=0 ("disabled index (row)"), index (col) #1=0 ("disabled index (col)"), new element #2=w285, index (row) #2=0 ("disabled index (row)"), index (col) #2=2 ("disabled index (col)")) -> (w286:string[][])
        n181 = property on="Schedule" class="MCListbox (strict)"("ItemNames"=w286) -> ()  [unwired: 2 in, 2 out]
      }
      frame "Insert" {
        w292 = ".........."
        n182 = property on="Schedule" class="MCListbox (strict)"() -> ("FocusRow"=w300:i32)  [unwired: 2 in, 2 out]
        n183 = Initialize Array("0.00000", 19 ("dimension size")) -> (w297:string[])
        n184 = Initialize Array(w292, 2 ("dimension size")) -> (w296:string[])
        n185 = property on="Schedule" class="MCListbox (strict)"() -> ("ItemNames"=w295:string[][])  [unwired: 2 in, 2 out]
        n186 = Initialize Array(w292, 21 ("dimension size")) -> (w298:string[])
        n187 = Replace Array Subset(array=w298, new element #1=w296, index #1=0 ("index"), new element #2=w297, index #2=2 ("index")) -> (w299:string[])
        n188 = Insert Into Array(array=w295, index (row)=w300, new element=w299) -> (w301:string[][])  [unwired: 1 in]
        n189 = property on="Schedule" class="MCListbox (strict)"("ItemNames"=w301) -> ()  [unwired: 2 in, 2 out]
      }
      frame "Delete" {
        w307 = ".........."
        n190 = property on="Schedule" class="MCListbox (strict)"() -> ("FocusRow"=w320:i32)  [unwired: 2 in, 2 out]
        n191 = Initialize Array("0.00000", 19 ("dimension size")) -> (w313:string[])
        n192 = Initialize Array(w307, 2 ("dimension size")) -> (w312:string[])
        n193 = Initialize Array("") -> ()  [unwired: 1 in, 1 out]
        n194 = property on="Schedule" class="MCListbox (strict)"() -> ("ItemNames"=w317:string[][])  [unwired: 2 in, 2 out]
        n195 = Initialize Array(w307, 21 ("dimension size")) -> (w314:string[])
        n196 = Replace Array Subset(array=w314, new element #1=w312, index #1=0 ("index"), new element #2=w313, index #2=2 ("index")) -> (w315:string[])
        n197 = Delete From Array(array=w317, index (row)=w320) -> (deleted portion=w319:string[], array with subset deleted=w318:string[][])  [unwired: 2 in]
        n198 = property on="Copied Row" class="Arr (strict)"("Value"=w319) -> ()  [unwired: 2 in, 2 out]
        n199 = Insert Into Array(array=w318, index (row)=31, new element=w315) -> (w316:string[][])  [unwired: 1 in]
        n200 = property on="Schedule" class="MCListbox (strict)"("ItemNames"=w316) -> ()  [unwired: 2 in, 2 out]
      }
      frame "Copy" {
        n201 = property on="Schedule" class="MCListbox (strict)"() -> ("ItemNames"=w322:string[][])  [unwired: 2 in, 2 out]
        n202 = property on="Schedule" class="MCListbox (strict)"() -> ("FocusRow"=w323:i32)  [unwired: 2 in, 2 out]
        n203 = Index Array(array=w322, index (row)=w323) -> (element=w324:string[])  [unwired: 1 in]
        n204 = property on="Copied Row" class="Arr (strict)"("Value"=w324) -> ()  [unwired: 2 in, 2 out]
      }
      frame "Paste" {
        n205 = property on="Schedule" class="MCListbox (strict)"() -> ("FocusRow"=w330:i32)  [unwired: 2 in, 2 out]
        n206 = property on="Copied Row" class="Arr (strict)"() -> ("Value"=w329:string[])  [unwired: 2 in, 2 out]
        n207 = property on="Schedule" class="MCListbox (strict)"() -> ("ItemNames"=w328:string[][])  [unwired: 2 in, 2 out]
        n208 = Array Size(array=w329) -> (size(s)=w326:i32)
        n209 = Greater Than 0?(x=w326) -> (x > 0?=w327:bool)
        n210 = case shown="True" w327 {
          tunnel: w328 -> [_ w334]
          tunnel: w329 -> [_ w333]
          tunnel: w330 -> [_ w332]
          frame False {
          }
          frame True {
            n211 = Replace Array Subset(array=w334, new element=w333, index (row)=w332) -> (w331:string[][])  [unwired: 1 in]
            n212 = property on="Schedule" class="MCListbox (strict)"("ItemNames"=w331) -> ()  [unwired: 2 in, 2 out]
          }
        }
      }
      frame "Save Sched" {
        n213 = property on="Schedule Name" class="Str"() -> ("Value"=w352:string)  [unwired: 2 in, 2 out]
        n214 = property on="SchedNames[]" class="Arr (strict)"() -> ("Value"=w351:string[])  [unwired: 2 in, 2 out]
        n215 = property on="Sched#" class="Ring (strict)"() -> ("Value"=w354:u16)  [unwired: 2 in, 2 out]
        n216 = property on="Schedule" class="MCListbox (strict)"() -> ("ItemNames"=w347:string[][])  [unwired: 2 in, 2 out]
        n217 = Decrement(x=w354) -> (x-1=w353:u16)
        n218 = Replace Array Subset(array=w351, new element=w352, index=w353) -> (w355:string[])
        n219 = Array Subset(array=w347, index (row)=0 ("index"), length (row)=32 ("length"), index (col)=0 ("index"), length (col)=21 ("length")) -> (w348:string[][])
        n220 = Number To Decimal String(number=w354) -> (decimal integer string=w349:string)  [unwired: 1 in]
        n221 = call <vilib>:"1D String Array to Delimited String.vi"("delimiter"=",\n", "string array"=w355) -> ("delimited string"=w356:string)  [unwired: 9 in]
        n222 = Concatenate Strings("Sched" ("File Save As"), w349) -> (w350:string)
        n223 = Transpose 2D Array(2D array=w348) -> (transposed array=w346:string[][])
        n224 = Reshape Array(w346, 672 ("dimension size")) -> (w345:string[])
        n225 = Write to Text File(file (use dialog)=path "C:/Users/Public/Documents/Grid2093/SCHEDS/SchedNames.txt" ("path"), text=w356) -> ()  [unwired: 2 in, 3 out]
        n226 = call "XML Write Scheds.vi"("error in"=w336, "File Save As"=w350, "Sched Values"=w345) -> ("error out"=w335:errorcluster)  [unwired: 8 in]
      }
      frame "Load Step Vals" {
        n227 = property on="Schedule" class="MCListbox (strict)"() -> ("ItemNames"=w359:string[][])  [unwired: 2 in, 2 out]
        n228 = property on="Schedule" class="MCListbox (strict)"() -> ("FocusRow"=w363:i32)  [unwired: 2 in, 2 out]
        n229 = Index Array(array=w359, index (row)=w363) -> (element=w358:string[])  [unwired: 1 in]
        n230 = call "StepVals.vi"("Step Array"=w358) -> ("SAVED"=w361:bool, "output array"=w362:string[], "DONE"=w360:bool)  [unwired: 8 in]
        n231 = case shown="True" w360 {
          tunnel: w361 -> [_ w366]
          tunnel: w362 -> [_ w365]
          tunnel: w363 -> [_ w364]
          frame False {
          }
          frame True {
            n232 = case shown="True" w366 {
              tunnel: w365 -> [_ w369]
              tunnel: w364 -> [_ w370]
              frame False {
              }
              frame True {
                n233 = property on="Schedule" class="MCListbox (strict)"() -> ("ItemNames"=w368:string[][])  [unwired: 2 in, 2 out]
                n234 = Replace Array Subset(array=w368, new element=w369, index (row)=w370) -> (w371:string[][])  [unwired: 1 in]
                n235 = property on="Schedule" class="MCListbox (strict)"("ItemNames"=w371) -> ()  [unwired: 2 in, 2 out]
              }
            }
            n236 = property on="LOAD STEP VAL" class="Bool (strict)"("Value"=FALSE ("LOAD STEP VAL")) -> ()  [unwired: 2 in, 2 out]
          }
        }
      }
      frame "Exit" {
        n237 = call "Flush Message Queue.vi"("Error In"=w375) -> ("Error Out"=w374:errorcluster)  [unwired: 9 in, 1 out]
        n238 = property on="Tab Control" class="TabCtl (strict)"("Value"=enum32{"Schedule", "Tubes"}."Schedule" ("Tab Control")) -> ()  [unwired: 2 in, 2 out]
      }
      frame "Tubes Tab" {
        w376 = 0 ("Focus Row")
        n239 = call "XML Parser Tubes.vi"("error in (no error)"=w383) -> ("error out"=w389:errorcluster, "output array"=w388:string[])  [unwired: 9 in]
        n240 = Reshape Array(w388, 9 ("dimension size"), 31 ("dimension size")) -> (w387:string[][])
        n241 = Transpose 2D Array(2D array=w387) -> (transposed array=w386:string[][])
        n242 = property on="Tube Type" class="MCListbox (strict)"(error in=w389, "ItemNames"=w386) -> (error out=w382:errorcluster)  [unwired: 1 in, 1 out]
        n243 = property on="Tube Type" class="MCListbox (strict)"(error in=w382, "FocusRow"=w376) -> (error out=w378:errorcluster)  [unwired: 1 in, 1 out]
        n244 = To Variant(anything=w376) -> (Variant=w379:variant)
        n245 = call "Enqueue Message (Single).vi"("Error In"=w378, "Message Position"=Message_Queue_Element_Position."Back", "Data"=w379, "State Machine Message"=State_Machine_Message."Tube Select") -> ("Error Out"=w377:errorcluster)  [unwired: 7 in]
      }
      frame "Tube Select" {
        w405 = u32 0 ("default (0 I32)")
        n246 = property on="Tube Type" class="MCListbox (strict)"() -> ("FocusRow"=w393:i32)  [unwired: 2 in, 2 out]
        n247 = Variant To Data(error in=w395, type=w393, Variant=w394) -> (data=w392:i32, error out=w391:errorcluster)
        n248 = property on="Tube Type" class="MCListbox (strict)"() -> ("ItemNames"=w406:string[][])  [unwired: 2 in, 2 out]
        n249 = Index Array(array=w406, index (row) #1=w392, index (col) #1=0 ("disabled index (col)"), index (row) #2=w392, index (col) #2=1 ("disabled index (col)"), index (row) #3=w392, index (col) #3=2 ("disabled index (col)"), index (row) #4=w392, index (col) #4=3 ("disabled index (col)"), index (row) #5=w392, index (col) #5=4 ("disabled index (col)"), index (row) #6=w392, index (col) #6=5 ("disabled index (col)"), index (row) #7=w392, index (col) #7=6 ("disabled index (col)"), index (row) #8=w392, index (col) #8=7 ("disabled index (col)"), index (row) #9=w392, index (col) #9=8 ("disabled index (col)")) -> (element #1=w407:string, element #2=w408:string, element #3=w410:string, element #4=w415:string, element #5=w416:string, element #6=w417:string, element #7=w418:string, element #8=w419:string, element #9=w420:string)
        n250 = Decimal String To Number(string=w418, default (0L)=w405) -> (number=w421:u32)  [unwired: 1 in, 1 out]
        n251 = Decimal String To Number(string=w408) -> (number=w409:i32)  [unwired: 2 in, 1 out]
        n252 = Decimal String To Number(string=w410) -> (number=w411:i32)  [unwired: 2 in, 1 out]
        n253 = Decimal String To Number(string=w415) -> (number=w412:i32)  [unwired: 2 in, 1 out]
        n254 = Decimal String To Number(string=w416) -> (number=w413:i32)  [unwired: 2 in, 1 out]
        n255 = Decimal String To Number(string=w419, default (0L)=w405) -> (number=w427:u32)  [unwired: 1 in, 1 out]
        n256 = Decimal String To Number(string=w417) -> (number=w414:i32)  [unwired: 2 in, 1 out]
        n257 = Decimal String To Number(string=w420, default (0L)=w405) -> (number=w428:u32)  [unwired: 1 in, 1 out]
        n258 = Number To Boolean Array(number=w427) -> (Boolean array=w425:bool[])
        n259 = Number To Boolean Array(number=w428) -> (Boolean array=w426:bool[])
        n260 = Number To Boolean Array(number=w421) -> (Boolean array=w422:bool[])
        n261 = Bundle By Name(cluster=T5 {"Tube Name"="Check", "T0"=85.0, "RTC"=340.0, "HS"=3700.0, "T100"=1085.0, "AP%"=70.0} ("Tube Values"), "Tube Name"=w407, "RTC"=w409, "HS"=w411, "T100"=w412, "T0"=w413, "AP%"=w414) -> (w423:T5)
        n262 = Array To Cluster(array=w425) -> (cluster=w429:T8)
        n263 = Array To Cluster(array=w426) -> (cluster=w430:T8)
        n264 = Array To Cluster(array=w422) -> (cluster=w424:T8)
        n265 = property on="Sched 1-30" class="Clust (strict)"("Value"=w424) -> ()  [unwired: 2 in, 2 out]
        n266 = property on="Sched 31-60" class="Clust (strict)"("Value"=w429) -> ()  [unwired: 2 in, 2 out]
        n267 = property on="Sched 61-80" class="Clust (strict)"("Value"=w430) -> ()  [unwired: 2 in, 2 out]
        n268 = property on="Tube Values" class="Clust (strict)"("Value"=w423) -> ()  [unwired: 2 in, 2 out]
      }
      frame "Tube Save" {
        n269 = property on="Tube Values" class="Clust (strict)"() -> ("Value"=w459:T5)  [unwired: 2 in, 2 out]
        n270 = property on="Sched 1-30" class="Clust (strict)"() -> ("Value"=w442:T3)  [unwired: 2 in, 2 out]
        n271 = property on="Sched 31-60" class="Clust (strict)"() -> ("Value"=w441:T3)  [unwired: 2 in, 2 out]
        n272 = property on="Sched 61-80" class="Clust (strict)"() -> ("Value"=w440:T3)  [unwired: 2 in, 2 out]
        n273 = Unbundle By Name(w459) -> ("Tube Name"=w452:string, "RTC"=w458:dbl, "HS"=w454:dbl, "T100"=w457:dbl, "T0"=w456:dbl, "AP%"=w455:dbl)
        n274 = Cluster To Array(cluster=w440) -> (array=w437:bool[])
        n275 = Cluster To Array(cluster=w442) -> (array=w439:bool[])
        n276 = Cluster To Array(cluster=w441) -> (array=w438:bool[])
        n277 = Boolean Array To Number(Boolean array=w439) -> (number=w436:u32)
        n278 = Boolean Array To Number(Boolean array=w438) -> (number=w435:u32)
        n279 = Boolean Array To Number(Boolean array=w437) -> (number=w434:u32)
        n280 = property on="Tube Type" class="MCListbox (strict)"() -> ("ItemNames"=w443:string[][])  [unwired: 2 in, 2 out]
        n281 = Number To Decimal String(number=w435) -> (decimal integer string=w431:string)  [unwired: 1 in]
        n282 = Number To Decimal String(number=w458) -> (decimal integer string=w453:string)  [unwired: 1 in]
        n283 = Number To Decimal String(number=w454) -> (decimal integer string=w451:string)  [unwired: 1 in]
        n284 = Number To Decimal String(number=w457) -> (decimal integer string=w450:string)  [unwired: 1 in]
        n285 = Number To Decimal String(number=w456) -> (decimal integer string=w449:string)  [unwired: 1 in]
        n286 = Number To Decimal String(number=w455) -> (decimal integer string=w448:string)  [unwired: 1 in]
        n287 = Number To Decimal String(number=w434) -> (decimal integer string=w432:string)  [unwired: 1 in]
        n288 = Number To Decimal String(number=w436) -> (decimal integer string=w433:string)  [unwired: 1 in]
        n289 = property on="Tube Type" class="MCListbox (strict)"() -> ("FocusRow"=w446:i32)  [unwired: 2 in, 2 out]
        n290 = Build Array(w452, w453, w451, w450, w449, w448, w433, w431, w432) -> (w447:string[])
        n291 = Replace Array Subset(array=w443, new element=w447, index (row)=w446) -> (w444:string[][])  [unwired: 1 in]
        n292 = property on="Tube Type" class="MCListbox (strict)"("ItemNames"=w444) -> ()  [unwired: 2 in, 2 out]
        n293 = Transpose 2D Array(2D array=w444) -> (transposed array=w463:string[][])
        n294 = Reshape Array(w463, 279 ("dimension size")) -> (w445:string[])
        n295 = call "XML Write Tubes.vi"("error in"=w461, "Tube Values"=w445) -> ("error out"=w460:errorcluster)  [unwired: 8 in, 1 out]
      }
    }
    n296 = call "Enqueue Handle Error Message on Error.vi"("Error In"=w203) -> ("Error Out"=w202:errorcluster)  [unwired: 10 in]
  }
  n297 = Merge Errors(w6, w3) -> (w5:errorcluster)
  n298 = call "Destroy Message Queue.vi"("Error In"=w5) -> ("Error Out"=→"Error Out":errorcluster)  [unwired: 10 in]
